vi "FieldDisplaySmall.vi"() -> ()   [LabVIEW 2025]
uses:
  <vilib>/Rock Robotics/WPI/ThirdParty/JAS_Junk/TrajLib/TypeDef/FieldDisp_ElementPicture.ctl
  <vilib>/Rock Robotics/WPI/ThirdParty/JAS_Junk/TrajLib/Rotation2d_CreateAngle.vi
  <vilib>/Rock Robotics/WPI/ThirdParty/JAS_Junk/TrajLib/Translation2d_Create.vi
  <vilib>/Rock Robotics/WPI/ThirdParty/JAS_Junk/TrajLib/VI/FieldDisp_Element_Rotate.vi
  <vilib>/Rock Robotics/WPI/ThirdParty/JAS_Junk/TrajLib/Conv_Meters_Inches.vi
  <vilib>/Rock Robotics/WPI/ThirdParty/JAS_Junk/TrajLib/Conv_Radians_Deg.vi
  TargetCalcGlobals.vi
  <vilib>/picture/pixmap.llb/Flatten Pixmap.vi
  <vilib>/picture/pictutil.llb/Create Mask.vi
  <vilib>/picture/picture.llb/Draw Flattened Pixmap.vi
  <vilib>/Rock Robotics/WPI/ThirdParty/JAS_Junk/TrajLib/Trajectory_Library.lvlib
panel:
  out "ROBOT 2":T1
  out "Target Y M":dbl format="%11.2f"
  out "Target X M":dbl format="%11.2f"
  out "ROBOT":T1
  out "Robot Orient Rad":dbl format="%11.1f"
  out "Robot Y M":dbl format="%11.2f"
  out "Robot X M":dbl format="%11.2f"
  out "Field Picture":picture
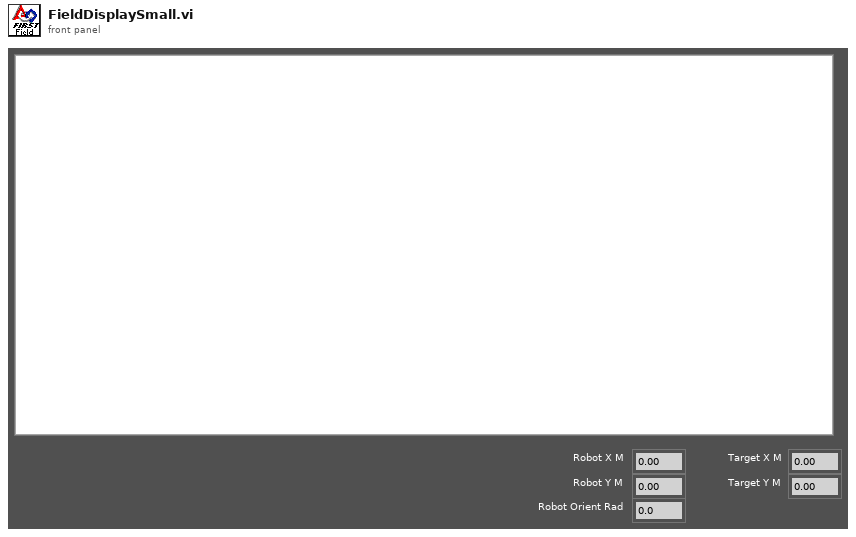
[diagram p1: front panel]
types:
  T1 = typedef "Trajectory_Library.lvlib/FieldDisp_ElementPicture.ctl" = picture
  T2 = typedef "Trajectory_Library.lvlib/FieldDisp_FieldElement.ctl" = cluster{"ONE-8-bit pixmap":u8[][], "Two-Array":cdb[][], "Three-Numeric":i32, "Four-Numeric":i32, "Five-Numeric":cdb, "Six-colors":u32[], "Seven-new element/subarray":u32, "Left Pixel":dbl, "Top Pixel":dbl, "Width Pix/Ft":dbl, "Height Pix/Ft":dbl, "Element Picture Ref":refnum<vi>}
  T3 = typedef "Trajectory_Library.lvlib/POSE2D.ctl" = cluster{"TRANSLATION":T4, "ROTATION":T5}
  T4 = typedef "Trajectory_Library.lvlib/TRANSLATION2D.ctl" = cluster{"X":dbl, "Y":dbl}
  T5 = typedef "Trajectory_Library.lvlib/ROTATION2D.ctl" = cluster{"VALUE":dbl, "COS":dbl, "SIN":dbl}
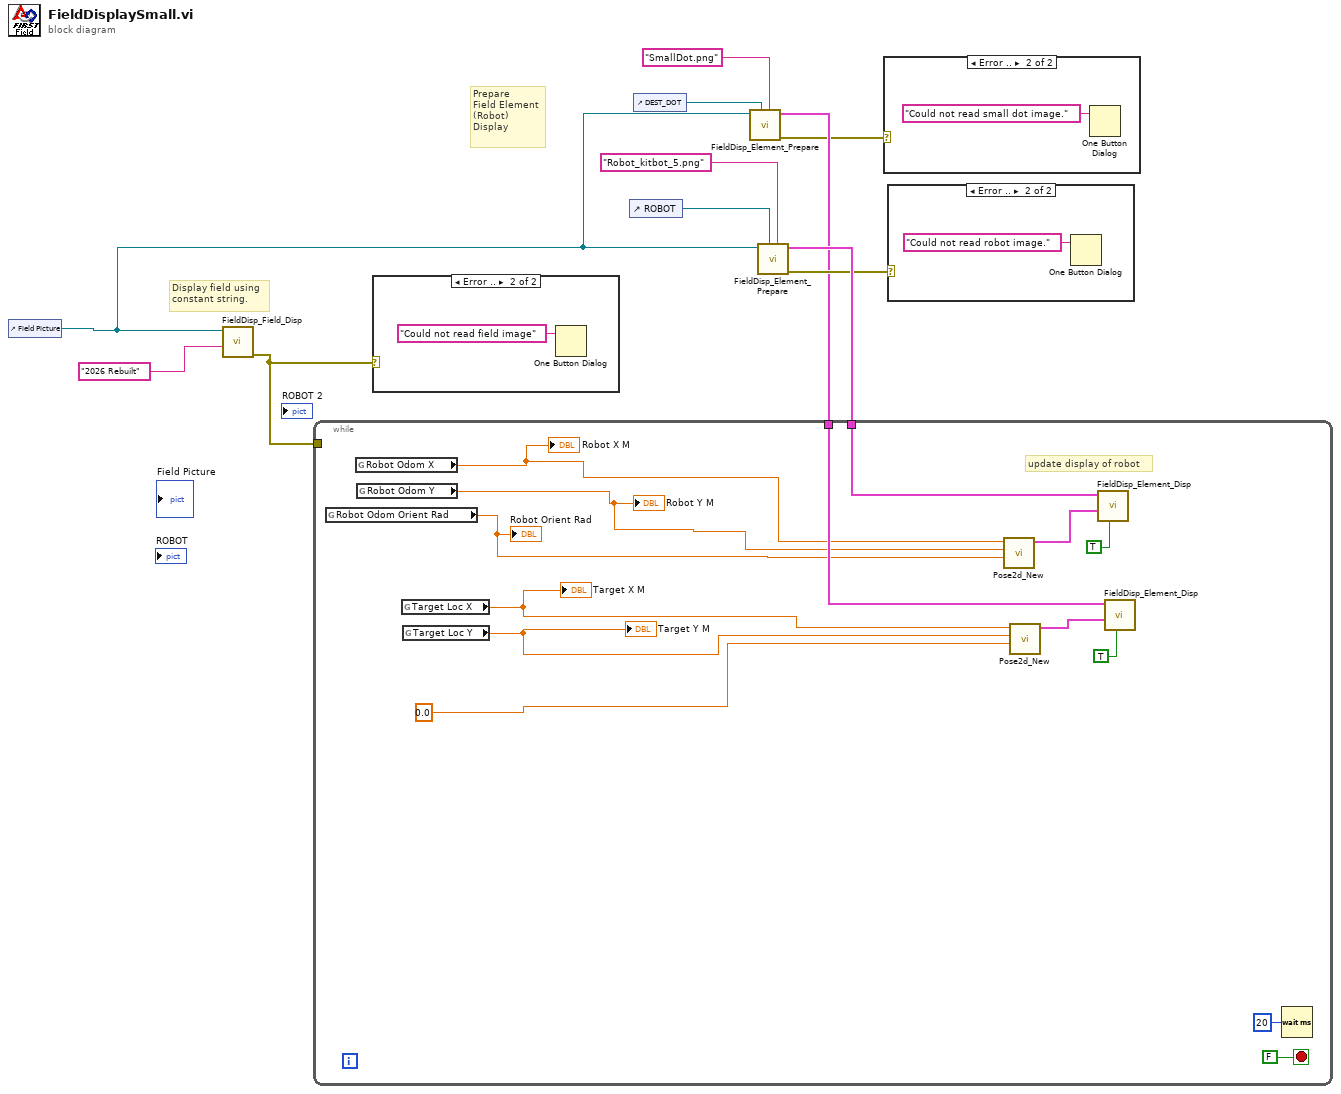
[diagram p0: block diagram]
diagram:
  # "Prepare\nField Element\n(Robot)\nDisplay"
  # "Display field using\nconstant string."
  n1 = control-ref of="Field Picture"() -> (w3:refnum<vi>)
  n2 = call <vilib>:"FieldDisp_Field_Disp.vi"("Field Selector"="2026 Rebuilt", "Picture in"=w3) -> ("error out"=w6:errorcluster)  [unwired: 9 in]
  n3 = case shown="Error .." w6 {
    frame No Error {
    }
    frame Error {
      n4 = One Button Dialog(message="Could not read field image") -> ()  [unwired: 1 in, 1 out]
    }
  }
  n5 = control-ref of="ROBOT"() -> (w9:refnum<vi>)
  n6 = control-ref of="DEST_DOT"() -> (w5:refnum<vi>)
  n7 = call <vilib>:"FieldDisp_Element_Prepare.vi"("Element File Name"="SmallDot.png" ("Picture FIle Name"), "Element Picture Ref"=w5, "Field Picture Ref"=w3) -> ("error out"=w1:errorcluster, "Field Element Info"=w2:T2)  [unwired: 7 in]
  n8 = call <vilib>:"FieldDisp_Element_Prepare.vi"("Element File Name"="Robot_kitbot_5.png" ("Picture FIle Name"), "Element Picture Ref"=w9, "Field Picture Ref"=w3) -> ("error out"=w7:errorcluster, "Field Element Info"=w8:T2)  [unwired: 7 in]
  n9 = while {
    tunnel: w8 -> [w25]
    tunnel: w6 -> [_]
    tunnel: w2 -> [w20]
    stop <- FALSE stop-if-true
    # "update display of robot"
    n10 = global read "TargetCalcGlobals.vi" "Robot Odom Orient Rad"() -> (w16:dbl)
    "Robot Orient Rad" <- w16
    n11 = global read "TargetCalcGlobals.vi" "Robot Odom X"() -> (w18:dbl)
    "Robot X M" <- w18
    n12 = global read "TargetCalcGlobals.vi" "Robot Odom Y"() -> (w17:dbl)
    "Robot Y M" <- w17
    n13 = global read "TargetCalcGlobals.vi" "Target Loc X"() -> (w14:dbl)
    "Target X M" <- w14
    n14 = global read "TargetCalcGlobals.vi" "Target Loc Y"() -> (w13:dbl)
    "Target Y M" <- w13
    n15 = call <vilib>:"Pose2d_New.vi"("Heading"=w16, "Y"=w17, "X"=w18) -> ("out POSe"=w24:T3)  [unwired: 8 in]
    n16 = call <vilib>:"Pose2d_New.vi"("Heading"=0.0, "Y"=w13, "X"=w14) -> ("out POSe"=w19:T3)  [unwired: 8 in]
    n17 = call <vilib>:"FieldDisp_Element_Disp.vi"("Visible"=TRUE, "Element Pose"=w24, "Element Info"=w25) -> ()  [unwired: 9 in]
    n18 = call <vilib>:"FieldDisp_Element_Disp.vi"("Visible"=TRUE, "Element Pose"=w19, "Element Info"=w20) -> ()  [unwired: 9 in]
    n19 = Wait (ms)(milliseconds to wait=u32 20) -> ()  [unwired: 1 out]
  }
  n20 = case shown="Error .." w1 {
    frame No Error {
    }
    frame Error {
      n21 = One Button Dialog(message="Could not read small dot image.") -> ()  [unwired: 1 in, 1 out]
    }
  }
  n22 = case shown="Error .." w7 {
    frame No Error {
    }
    frame Error {
      n23 = One Button Dialog(message="Could not read robot image.") -> ()  [unwired: 1 in, 1 out]
    }
  }
